vi "Extract DPs and Noise.vi"(0 "DataAcq":T2, 1 "DP Freqs":T1, 5 "Spectrum in Vrms":dbl[](array[numeric]) format="%.8f", 9 "Phase":dbl[](array[numeric]), 11 "SPL":dbl) -> (8 "Output Array":dbl[](array[numeric]))   [LabVIEW 2020]
uses:
  Typedefs/DP-DataAcq.ctl
  Typedefs/DP-Freqs.ctl
  epl-vi-lib/Utility VIs/Math VIs/Linear to dB (scalar).vi
panel:
  # "SPL\nf1 (Hz)\nf2 (Hz)\nf1\nf2\n2f1-f2\nNse 2f1-f2\nf2-f1\nNse f2-f1\nPhase 2f1-f2"
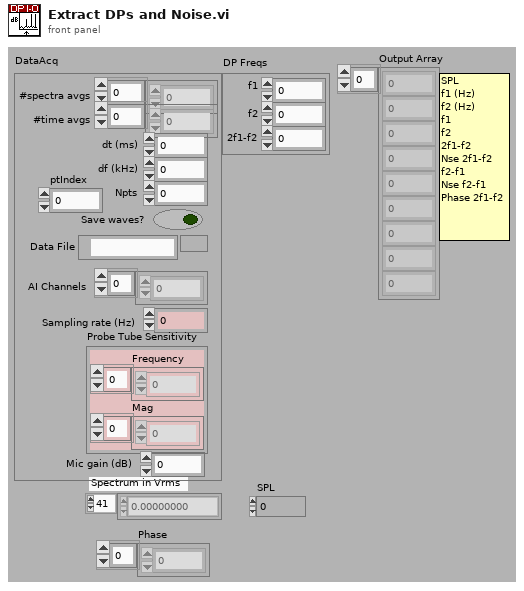
[diagram p1: front panel]
types:
  T1 = typedef "DP-Freqs.ctl" = cluster{"f1":dbl, "f2":dbl, "2f1-f2":dbl}
  T2 = typedef "DP-DataAcq.ctl" = cluster{"#spectra avgs":i32[], "#time avgs":i32[], "dt (ms)":dbl, "df (kHz)":dbl, "Npts":i32, "Save waves?":bool, "Data File":path, "AI Channels":u16[], "Sampling rate (Hz)":dbl, "Probe Tube Sensitivity":cluster{"Frequency":dbl[], "Mag":dbl[]}, "Mic gain (dB)":dbl, "ptIndex":i32}
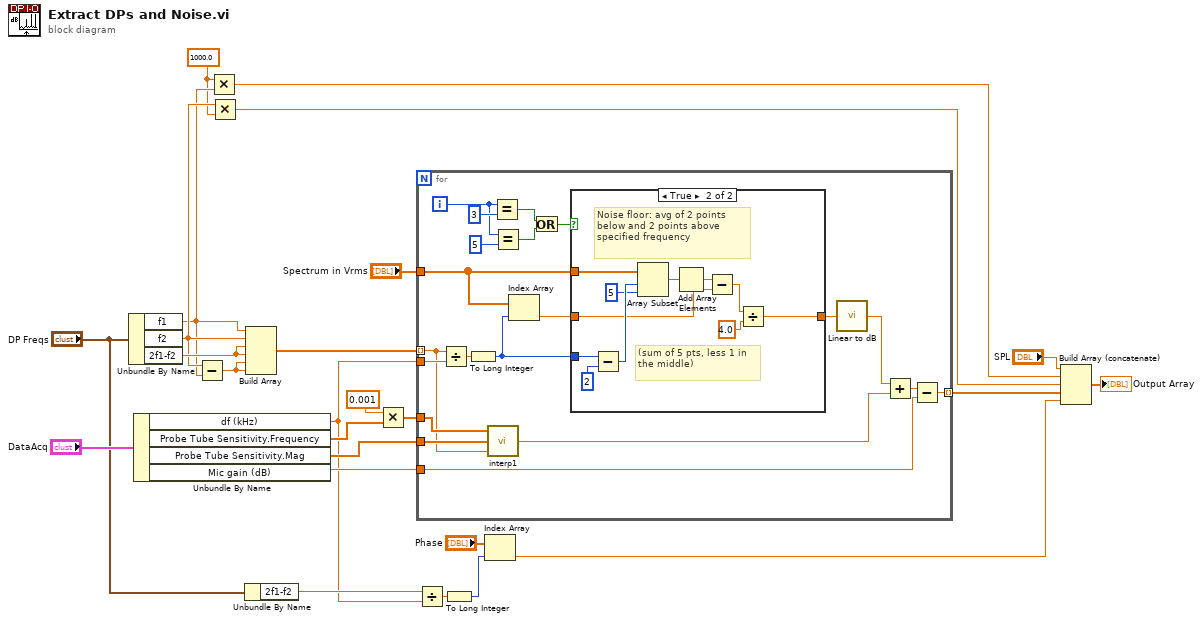
[diagram p0: block diagram]
diagram:
  w8 = 1000.0
  n1 = Unbundle By Name("DP Freqs") -> ("f1"=w10:dbl, "f2"=w13:dbl, "2f1-f2"=w18:dbl)
  n2 = Unbundle By Name("DataAcq") -> ("df (kHz)"=w3:dbl, "Probe Tube Sensitivity.Frequency"=w22:dbl[], "Probe Tube Sensitivity.Mag"=w21:dbl[], "Mic gain (dB)"=w12:dbl)
  n3 = Subtract(x=w13, y=w10) -> (x-y=w17:dbl)
  n4 = Multiply(x=w8, y=w10) -> (x*y=w11:dbl)
  n5 = Multiply(x=w13, y=w8) -> (x*y=w9:dbl)
  n6 = Unbundle By Name("DP Freqs") -> ("2f1-f2"=w4:dbl)
  n7 = Build Array(w10, w13, w18, w18, w17, w17) -> (w16:dbl[])
  n8 = Multiply(x=0.001, y=w22) -> (x*y=w25:dbl[])
  n9 = for {
    tunnel: w21 -> [w42]
    tunnel: [w45] -> w14 mode=indexing
    tunnel: w25 -> [w43]
    tunnel: w12 -> [w39]
    tunnel: w16 -> [w36] mode=indexing
    tunnel: "Spectrum in Vrms" -> [w26]
    tunnel: w3 -> [w38]
    i -> [w34]
    n10 = Divide(x=w36, y=w38) -> (x/y=w37:dbl)
    n11 = To Long Integer(number=w37) -> (32bit integer=w28:i32)
    n12 = call "interp1.vi"("X"=w43, "Y"=w42, "U"=w36) -> ("V"=w40:dbl)  [unwired: 2 in]
    n13 = Equal?(x=w34, y=3) -> (x = y?=w31:bool)
    n14 = Equal?(x=w34, y=5) -> (x = y?=w30:bool)
    n15 = Index Array(array=w26, index=w28) -> (element=w29:dbl)
    n16 = Or(x=w31, y=w30) -> (x .or. y?=w32:bool)
    n17 = case shown="True" w32 {
      tunnel: w29 -> [w46 w52]
      tunnel: w28 -> [_ w57]
      tunnel: [w46 w47] -> w27
      tunnel: w26 -> [_ w48]
      frame False {
      }
      frame True {
        # "(sum of 5 pts, less 1 in the middle)"
        # "Noise floor: avg of 2 points\nbelow and 2 points above specified frequency"
        n18 = Subtract(x=w57, y=2) -> (x-y=w55:i32)
        n19 = Array Subset(array=w48, index=w55, length=5) -> (w53:dbl[])
        n20 = Add Array Elements(numeric array=w53) -> (sum=w49:dbl)
        n21 = Subtract(x=w49, y=w52) -> (x-y=w51:dbl)
        n22 = Divide(x=w51, y=4.0) -> (x/y=w47:dbl)
      }
    }
    n23 = call-poly "Linear to dB.vi"("Linear"=w27) -> ("dB"=w41:dbl)
    n24 = Add(x=w41, y=w40) -> (x+y=w44:dbl)
    n25 = Subtract(x=w44, y=w39) -> (x-y=w45:dbl)
  }
  n26 = Divide(x=w4, y=w3) -> (x/y=w7:dbl)
  n27 = To Long Integer(number=w7) -> (32bit integer=w6:i32)
  n28 = Index Array(array="Phase", index=w6) -> (element=w1:dbl)
  n29 = Build Array (concatenate)("SPL", w11, w9, w14, w1) -> (→"Output Array":dbl[])
